vi "Reorganize_DB.vi"() -> ()   [LabVIEW 2013]
uses:
  <vilib>/Utility/miscctls.llb/LVPointTypeDef.ctl
  <userlib>/_OpenG.lib/file/file.llb/Valid Path - Traditional__ogtk.vi
  <userlib>/_OpenG.lib/array/array.llb/Search 1D Array (I32)__ogtk.vi
  <userlib>/_OpenG.lib/array/array.llb/Index 1D Array Elements (I32)__ogtk.vi
panel:
  out "file being worked on":i32
  out "Number of Files":i32
  out "Events that Errored":i32[](array[numeric])
  in  "Path":path
  out "error out":errorcluster
  in  "error in (no error)":errorcluster
  # "DO NOT RUN THIS PROGRAM unless you want to reorganize all .hdf5 files in the path above."
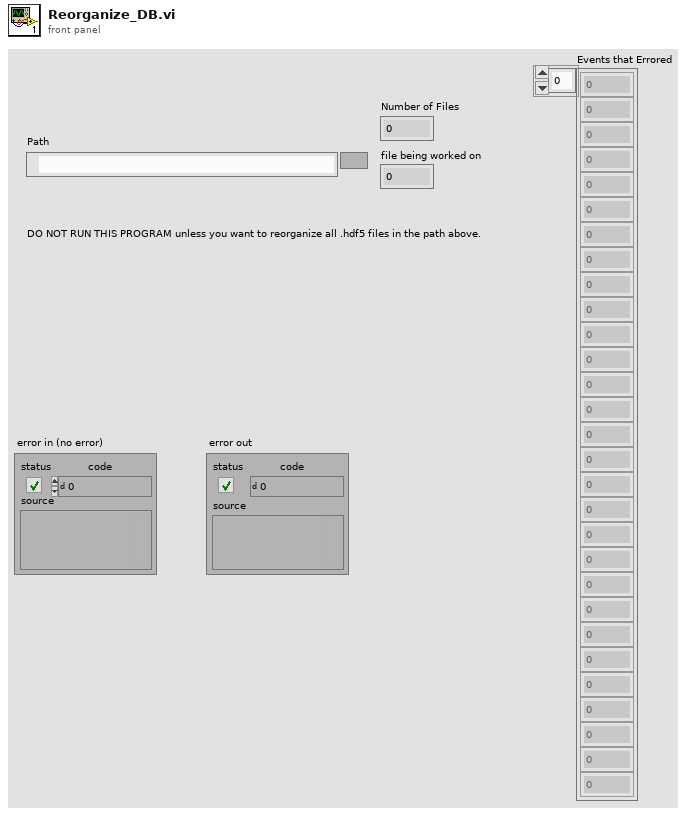
[diagram p1: front panel]
types:
  T1 = typedef "LVPointTypeDef.ctl" = cluster{"Horizontal":i16, "Vertical":i16}
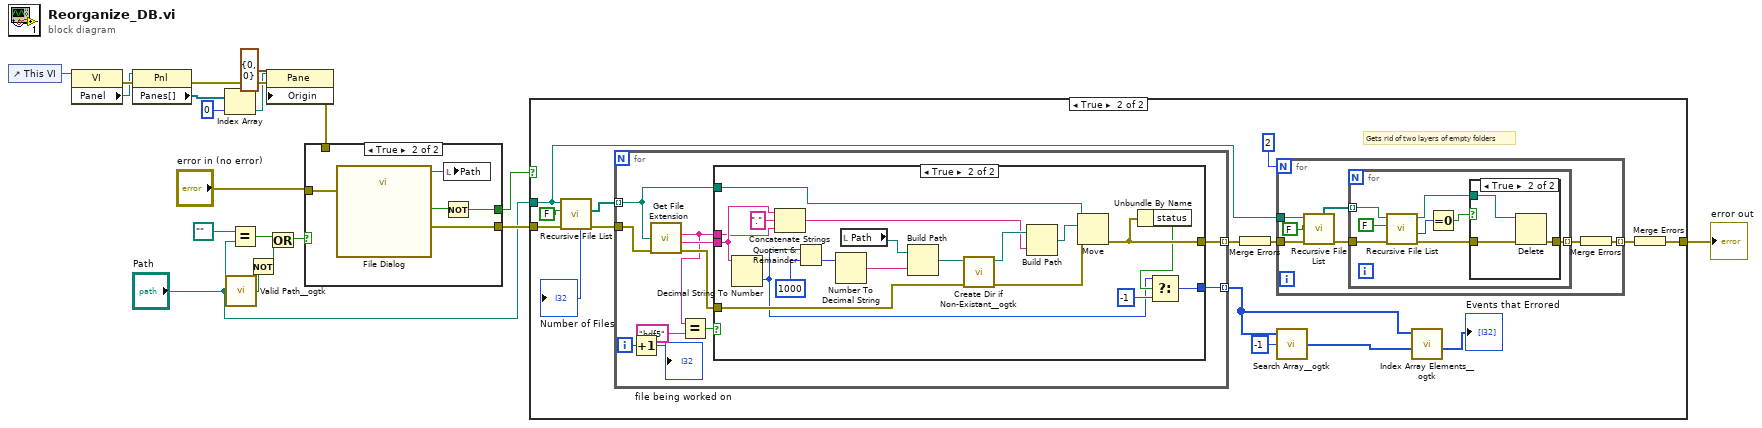
[diagram p0: block diagram]
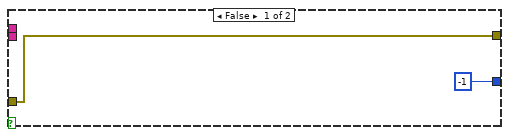
[diagram p3: hidden frame]
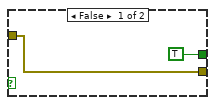
[diagram p5: hidden frame]
diagram:
  n1 = control-ref of="This VI"() -> (w19:refnum<vi>)
  n2 = property class="VI"(reference=w19) -> (error out=w18:errorcluster, "Panel"=w17:refnum<vi>)  [unwired: 1 in, 1 out]
  n3 = property class="Pnl"(reference=w17, error in=w18) -> (error out=w16:errorcluster, "Panes[]"=w15:refnum<vi>[])  [unwired: 1 out]
  n4 = Index Array(array=w15, index=0) -> (element=w13:refnum<vi>)
  n5 = call-poly <userlib>:"Valid Path__ogtk.vi"("path"="Path") -> ("valid"=w6:bool)
  n6 = Equal?(x=path "", y="Path") -> (x = y?=w10:bool)
  n7 = Not(x=w6) -> (.not. x?=w3:bool)
  n8 = property class="Pane"(reference=w13, error in=w16, "Origin"=T1 {"Horizontal"=0, "Vertical"=0}) -> (error out=w8:errorcluster)  [unwired: 1 out]
  n9 = Or(x=w10, y=w3) -> (x .or. y?=w7:bool)
  n10 = case shown="True" w7 {
    tunnel: [w21 w26] -> w5
    tunnel: "error in (no error)" -> [w21 w25]
    tunnel: w8 -> [_ _]
    tunnel: [TRUE w22] -> w1
    frame False {
    }
    frame True {
      n11 = call "File Dialog"("error in"=w25) -> ("selected path"=w24:path, "cancelled"=w23:bool, "error out"=w26:errorcluster)  [unwired: 11 in, 1 out]
      n12 = Not(x=w23) -> (.not. x?=w22:bool)
      n13 = local write "Path"(w24) -> ()
    }
  }
  n14 = case shown="True" w1 {
    tunnel: w5 -> [w27 w42]
    tunnel: "Path" -> [_ w30]
    tunnel: [w27 w34] -> w2
    frame False {
    }
    frame True {
      # "Gets rid of two layers of empty folders"
      n15 = call <vilib>:"Recursive File List.vi"("error in (no error)"=w42, "Treat LLBs as Folders?"=FALSE, "Folder Path"=w30) -> ("error out"=w40:errorcluster, "Number of Files"=→"Number of Files":i32, "All Files in Dir"=w39:path[])  [unwired: 4 in, 2 out]
      n16 = for {
        tunnel: w40 -> [w53]
        tunnel: w39 -> [w52] mode=indexing
        tunnel: [w50] -> w38 mode=indexing
        tunnel: [w49] -> w35 mode=indexing
        i -> [w44]
        n17 = Increment(x=w44) -> (x+1=→"file being worked on":i32)
        n18 = call <vilib>:"Get File Extension.vi"("error in (no error)"=w53, "file"=w52) -> ("error out"=w51:errorcluster, "filename without extension"=w47:string, "lowercase file extension"=w45:string)  [unwired: 6 in, 1 out]
        n19 = Equal?(x=w45, y="hdf5") -> (x = y?=w48:bool)
        n20 = case shown="True" w48 {
          tunnel: w47 -> [_ w66]
          tunnel: w45 -> [_ w65]
          tunnel: w52 -> [_ w64]
          tunnel: w51 -> [w55 w62]
          tunnel: [w55 w60] -> w50
          tunnel: [-1 ("f") w57] -> w49
          frame False {
          }
          frame True {
            n21 = Decimal String To Number(string=w66) -> (number=w56:i32)  [unwired: 2 in, 1 out]
            n22 = Concatenate Strings(w66, "." ("string"), w65) -> (w68:string)
            n23 = Quotient & Remainder(x=w56, y=1000) -> (floor(x/y)=w73:i32)  [unwired: 1 out]
            n24 = Number To Decimal String(number=w73) -> (decimal integer string=w61:string)  [unwired: 1 in]
            n25 = local read "Path"() -> (w72:path)
            n26 = Build Path(base path=w72, name or relative path=w61) -> (appended path=w71:path)
            n27 = call <userlib>:"Create Dir if Non-Existant__ogtk.vi"("error in (no error)"=w62, "Directory Path"=w71) -> ("error out"=w70:errorcluster, "dup Directory Path"=w69:path)  [unwired: 7 in, 1 out]
            n28 = Build Path(base path=w69, name or relative path=w68) -> (appended path=w63:path)
            n29 = Move(source path=w64, error in=w70, 10:w63) -> (error out=w60:errorcluster)  [unwired: 2 in, 2 out]
            n30 = Unbundle By Name(w60) -> ("status"=w59:bool)
            n31 = Select(t=w56, s=w59, f=-1) -> (s? t:f=w57:i32)
          }
        }
      }
      n32 = Merge Errors(w38) -> (w33:errorcluster)
      n33 = for {
        N: 2 -> [_]
        tunnel: [w80] -> w31 mode=indexing
        tunnel: w33 -> [w79]
        tunnel: w30 -> [w76]
        n34 = call <vilib>:"Recursive File List.vi"("error in (no error)"=w79, "Treat LLBs as Folders?"=FALSE, "Folder Path"=w76) -> ("error out"=w78:errorcluster, "All Folders"=w75:path[])  [unwired: 4 in, 3 out]
        n35 = for {
          tunnel: w78 -> [w85]
          tunnel: [w84] -> w81 mode=indexing
          tunnel: w75 -> [w82] mode=indexing
          n36 = call <vilib>:"Recursive File List.vi"("error in (no error)"=w85, "Treat LLBs as Folders?"=FALSE, "Folder Path"=w82) -> ("error out"=w86:errorcluster, "Number of Files"=w88:i32, "dup Folder Path"=w83:path)  [unwired: 4 in, 2 out]
          n37 = Equal To 0?(x=w88) -> (x = 0?=w87:bool)
          n38 = case shown="True" w87 {
            tunnel: w83 -> [_ w93]
            tunnel: w86 -> [w90 w92]
            tunnel: [w90 w91] -> w84
            frame False {
            }
            frame True {
              n39 = Delete(path (use dialog)=w93, error in=w92) -> (error out=w91:errorcluster)  [unwired: 3 in, 2 out]
            }
          }
        }
        n40 = Merge Errors(w81) -> (w80:errorcluster)
      }
      n41 = call-poly <userlib>:"Search Array__ogtk.vi"("Array"=w35, "Element Data"=-1) -> ("Indices of Elements"=w28:i32[])  [unwired: 7 in]
      n42 = call-poly <userlib>:"Index Array Elements__ogtk.vi"("indices"=w28, "array"=w35) -> ("elements"=→"Events that Errored":i32[])  [unwired: 9 in]
      n43 = Merge Errors(w31) -> (w34:errorcluster)
    }
  }
  "error out" <- w2
